vi "试剂余量后台任务.vi"   [LabVIEW 2016, in "斯坦道通用流路CODmn.lvlib"]
types:
  T1 = cluster{"V1":sgl, "V2":sgl, "V3":sgl, "V4":sgl, "V5":sgl, "V6":sgl, "V7":sgl, "V8":sgl, "V9":sgl, "V10":sgl, "V11":sgl, "V12":sgl, "V9-1":sgl, "V9-2":sgl}
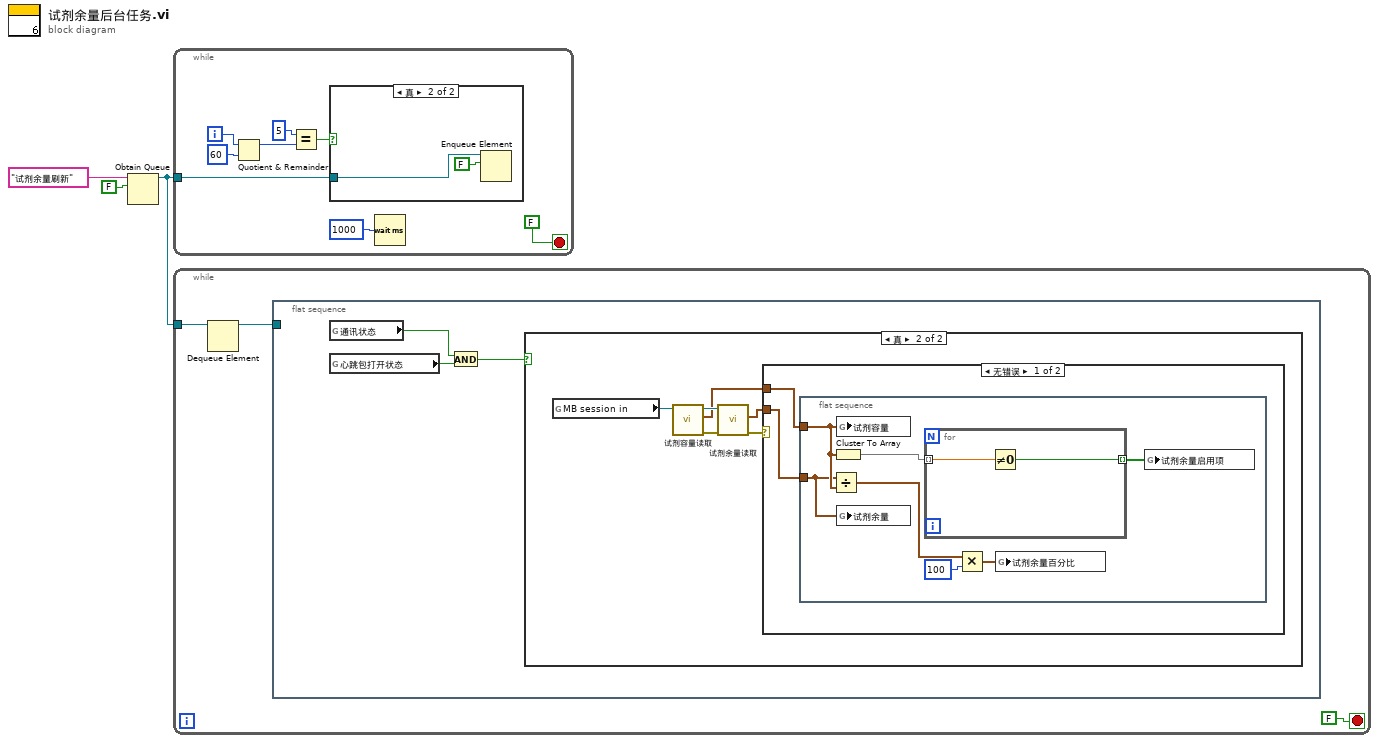
[diagram p0: block diagram]
diagram:
  n1 = Obtain Queue(name (unnamed)="试剂余量刷新" ("名称（未命名）"), element data type=FALSE) -> (queue out=w1:refnum<queue>)  [unwired: 3 in, 2 out]
  n2 = while {
    tunnel: w1 -> [w10]
    i -> [w8]
    stop <- FALSE stop-if-true
    n3 = Quotient & Remainder(x=w8, y=60) -> (x-y*floor(x/y)=w6:i32)  [unwired: 1 out]
    n4 = Equal?(x=5, y=w6) -> (x = y?=w5:bool)
    n5 = case shown="真" w5 {
      tunnel: w10 -> [_ w13]
      frame False {
      }
      frame True {
        n6 = Enqueue Element(queue=w13, element=FALSE ("元素")) -> ()  [unwired: 2 in, 3 out]
      }
    }
    n7 = Wait (ms)(milliseconds to wait=u32 1000 ("等待时间（毫秒）")) -> ()  [unwired: 1 out]
  }
  n8 = while {
    tunnel: w1 -> [w15]
    stop <- FALSE stop-if-true
    n9 = Dequeue Element(queue=w15) -> (queue out=w14:refnum<queue>)  [unwired: 2 in, 3 out]
    n10 = flat-sequence {
      tunnel: w14 -> [_]
      frame #0 {
        n11 = global read "VAR总磷总氮全局变量.vi" "通讯状态"() -> (w17:bool)
        n12 = global read "VAR总磷总氮全局变量.vi" "心跳包打开状态"() -> (w19:bool)
        n13 = And(x=w17, y=w19) -> (x .and. y?=w18:bool)
        n14 = case shown="真" w18 {
          frame False {
          }
          frame True {
            n15 = global read "VAR总磷总氮全局变量.vi" "MB session in"() -> (w23:refnum<class "MB_Master.lvclass">)
            n16 = call "试剂容量读取.vi"("MB session in"=w23) -> ("error out"=w25:errorcluster, "试剂容量"=w22:T1, "MB session out"=w24:refnum<class "MB_Master.lvclass">)  [unwired: 8 in]
            n17 = call "试剂余量读取.vi"("Error in"=w25, "MB session in"=w24) -> ("error out"=w20:errorcluster, "试剂余量"=w21:T1)  [unwired: 7 in, 1 out]
            n18 = case shown="无错误" w20 {
              tunnel: w22 -> [w27 _]
              tunnel: w21 -> [w26 _]
              frame No Error {
                n19 = flat-sequence {
                  tunnel: w27 -> [w32]
                  tunnel: w26 -> [w31]
                  frame #0 {
                    n20 = Divide(x=w31, y=w32) -> (x/y=w34:T1)
                    n21 = Cluster To Array(cluster=w32) -> (array=w29:sgl[])
                    n22 = global write "VAR总磷总氮全局变量.vi" "试剂容量"(w32) -> ()
                    n23 = global write "VAR总磷总氮全局变量.vi" "试剂余量"(w31) -> ()
                    n24 = for {
                      tunnel: w29 -> [w36] mode=indexing
                      tunnel: [w35] -> w28 mode=indexing
                      n25 = Not Equal To 0?(x=w36) -> (x != 0?=w35:bool)
                    }
                    n26 = Multiply(x=w34, y=100) -> (x*y=w30:T1)
                    n27 = global write "VAR总磷总氮全局变量.vi" "试剂余量百分比"(w30) -> ()
                    n28 = global write "VAR总磷总氮全局变量.vi" "试剂余量启用项"(w28) -> ()
                  }
                }
              }
              frame Error {
              }
            }
          }
        }
      }
    }
  }
